vi "PUMP_read_pressure.vi"(3 "error in":errorcluster, 4 "MFCS_EZ":T1, 5 "t0":dbl, 6 "Reset":bool) -> (0 "error out":errorcluster, 1 "Elapsed time (min/s)":u32, 2 "Pressure (mBar)":dbl)   [LabVIEW 2015]
uses:
  <userlib>/Fluigent/Fluigent MFCS/FluigentMFCS_Full.llb/_EZmfcsRefNum.ctl
  <userlib>/Fluigent/Fluigent MFCS/FluigentMFCS_Full.llb/_EZmfcsEnum.ctl
panel:
  out "Elapsed time (s)":u32
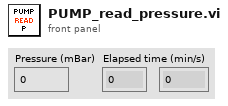
[diagram p1: front panel]
types:
  T1 = typedef "_EZmfcsRefNum.ctl" = refnum<k1>
  T2 = enum16{"Always On", "Always Off", "Off While Running"}
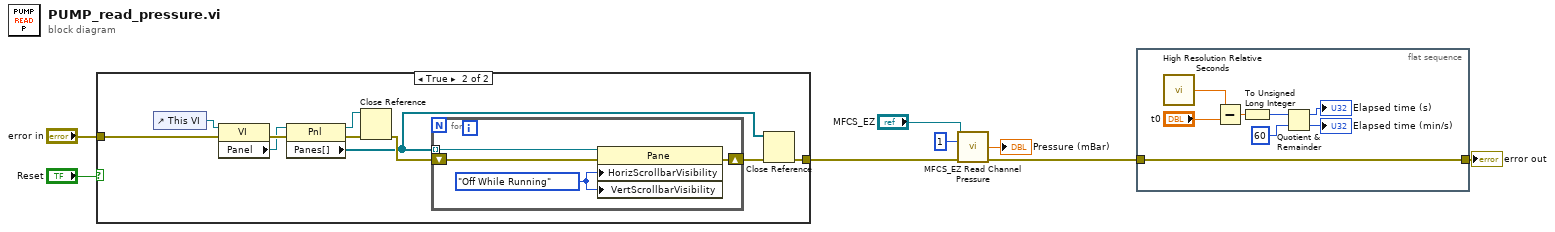
[diagram p0: block diagram]
diagram:
  n1 = case shown="True" "Reset" {
    tunnel: "error in" -> [w9 w11]
    tunnel: [w9 w10] -> w3
    frame False {
    }
    frame True {
      n2 = control-ref of="This VI"() -> (w12:refnum<vi>)
      n3 = property class="VI"(reference=w12, error in=w11) -> (error out=w14:errorcluster, "Panel"=w13:refnum<vi>)  [unwired: 1 out]
      n4 = property class="Pnl"(reference=w13, error in=w14) -> (reference out=w15:refnum<vi>, error out=w16:errorcluster, "Panes[]"=w18:refnum<vi>[])
      n5 = Close Reference(reference=w15, error in (no error)=w16) -> (error out=w19:errorcluster)
      n6 = for {
        tunnel: w18 -> [w23] mode=indexing
        shift-right: [w21] -> w17
        shift-left: w19 -> [w20]
        w22 = T2."Off While Running" ("Horizontal Scrollbar Visibility")
        n7 = property class="Pane"(reference=w23, error in=w20, "HorizScrollbarVisibility"=w22, "VertScrollbarVisibility"=w22) -> (error out=w21:errorcluster)  [unwired: 1 out]
      }
      n8 = Close Reference(reference=w18, error in (no error)=w17) -> (error out=w10:errorcluster)
    }
  }
  n9 = call <userlib>:"MFCS_EZ Read Channel Pressure.vi"("MFCS_EZ"="MFCS_EZ", "Channel Number (default=1)"=u8 1, "error in (no error)"=w3) -> ("Pressure (mBar)"=→"Pressure (mBar)":dbl, "error out"=w5:errorcluster)  [unwired: 9 in, 2 out]
  n10 = flat-sequence {
    tunnel: w5 -> [w28]
    tunnel: [w28] -> w4
    frame #0 {
      n11 = call <vilib>:"High Resolution Relative Seconds.vi"() -> ("relative seconds"=w31:dbl)
      n12 = Subtract(x=w31, y="t0") -> (x-y=w29:dbl)
      n13 = To Unsigned Long Integer(number=w29) -> (unsigned 32bit integer=w27:u32)
      n14 = Quotient & Remainder(x=w27, y=u32 60) -> (x-y*floor(x/y)=→"Elapsed time (s)":u32, floor(x/y)=→"Elapsed time (min/s)":u32)
    }
  }
  "error out" <- w4
